vi "TEST - Temporary Filename.vi"(8 "error in (no error)":errorcluster) -> (0 "error out":errorcluster, 2 "pass":bool)   [LabVIEW 2020]
uses:
  source/library/Valid Path/Valid Path - Traditional.vi
  <userlib>/_OpenG.lib/error/error.llb/openg_error.lvlib
  source/library/openg_file.lvlib
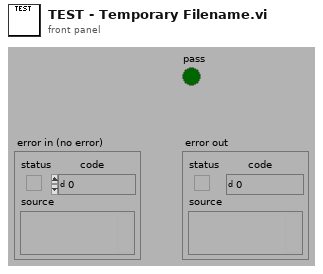
[diagram p1: front panel]
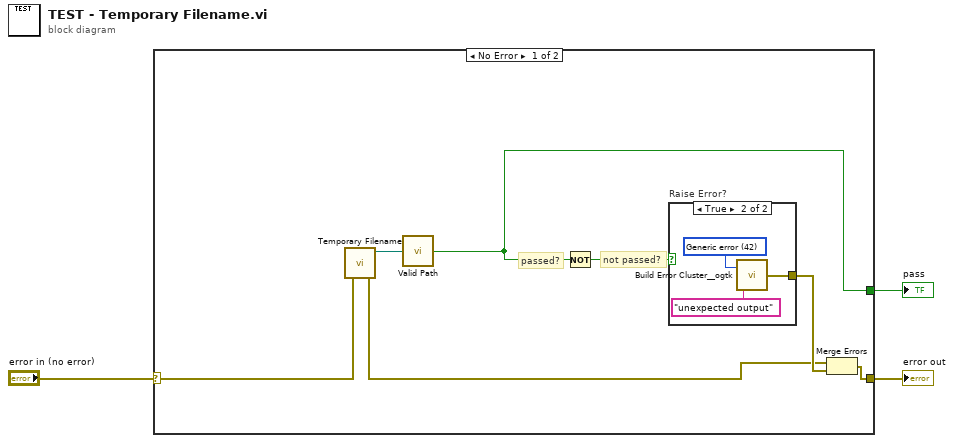
[diagram p0: block diagram]
diagram:
  n1 = case shown="No Error" "error in (no error)" {
    selector: "error in (no error)" -> [w6 w14]
    tunnel: [w4 _] -> w3
    tunnel: [w10 w14] -> w1
    frame No Error {
      # "not passed?"
      # "passed?"
      n2 = call "Temporary Filename.vi"("error in (no error)"=w6) -> ("error out"=w7:errorcluster, "file in tmp dir"=w5:path)  [unwired: 5 in]
      n3 = call-poly "Valid Path.vi"("path"=w5) -> ("valid"=w4:bool)
      n4 = Not(x=w4) -> (.not. x?=w8:bool)
      n5 = case "Raise Error?" shown="True" w8 {
        tunnel: [_ w11] -> w9
        frame False {
        }
        frame True {
          w12 = 42 items=["No error", "Argument error", "Memory is full", "Out of zone", "End of file", "File already open", "Generic file I/O error", "File not found", "File permission error", "Disk is full", "Duplicate path", "Too many files open", "System feature not enabled", "Resource file not found", "Cannot add resource", "Resource not found", "Image not found", "Image memory error", "Pen does not exist", "Config type invalid", "Config token not found", "Config parse error", "Config memory error", "Bad external code format", "Bad external code offset", "External code not present", "Null window", "Destroy window error", "Null menu", "Print aborted", "Bad print record", "Print driver error", "Windows error during printing", "Memory error during printing", "Print dialog error", "Generic print error", "Invalid device refnum", "Device not found", "Device parameter error", "Device unit error", "Cannot open device", "Device call aborted", "Generic error", "Cancelled by user", "Object ID too low", "Object ID too high", "Object not in heap", "Unknown heap", "Unknown object (invalid DefProc)", "Unknown object (DefProc not in table)", "Message out of range", "Invalid (null) method", "Unknown message", "Manager call not supported", "Bad address", "Network operation in progress", "Network operation timed out", "Connection is busy", "Network attribute not supported", "Network error", "Address in use", "System out of memory", "Connection aborted", "Connection refused", "Not connected", "Already connected", "Connection closed", "Initialization error (interapplication manager)", "Bad occurrence", "Wait on unbound occurrence handler", "Occurrence queue overflow", "Datalog type conflict", "Unused", "Unrecognized type (interapplication manager)", "Memory corrupt", "Failed to make temporary DLL", "Old CIN version", "Drag socket not found", "Failed to load drop-object", "Failed to register OLE object", "Failed to release OLE object", "Format specifier type mismatch", "Unknown format specifier", "Too few format specifiers", "Too many format specifiers", "Scan failed", "Newer CIN version", "Error converting to variant", "Runtime menu error", "Password tampered", "Variant attribute not found", "Incompatible variant data type", "Event data is not available", "Event Store is not present", "Occurrence is not found", "Event Queue is not created", "Event info is not available", "Refnum passed is NULL", "Error retrieving Class GUID", "Error retrieving CoClass GUID", "Error retrieving TypeLib GUID.", "Bad built application magic bytes.", "Specific driver is different from the specific driver associated with the Logical Name.", "There is no session opened to the class driver.", "Max Error", "MAX - Error with config objects", "MAX - Error loading configuration", "MAX - Group not supported"]
          n6 = call <userlib>:"Build Error Cluster__ogtk.vi"("String to Prepend to source (\"\")"="unexpected output" ("String to Prepend to source (\"\")"), "code"=w12) -> ("error out"=w11:errorcluster)
        }
      }
      n7 = Merge Errors(w7, w9) -> (w10:errorcluster)
    }
    frame Error {
    }
  }
  "pass" <- w3
  "error out" <- w1
